vi "Actor Teardown.vi"(10 "Error":errorcluster, 11 "Self Actor in":refnum<class "Self Actor.lvclass">) -> (0 "error out":errorcluster, 2 "Teardown?":bool, 3 "Self Actor out":refnum<class "Self Actor.lvclass">)   [LabVIEW 2021, in "LVCAM.lvlib" / "Self Actor.lvclass"]
uses:
  Self Actor.lvclass
  C:/PPLs/LabVIEW-Composed-Actor-Model-LVCAM/LabVIEW-Composed-Actor-Model-LVCAM/LVCAM/LVCAM/Actor/Actor.lvclass
  Self Actor.lvclass/Self Actor.ctl
  Msgs/Actor Destroy/Actor Destroy Msg Strategy/Actor Destroy Msg Strategy.lvclass
  C:/PPLs/LabVIEW-Composed-Actor-Model-LVCAM/LabVIEW-Composed-Actor-Model-LVCAM/LVCAM/LVCAM/Msg Strategy/Msg Strategy.lvclass
  Msgs/Actor Last Ack/Actor Last Ack Msg Strategy/Actor Last Ack Msg Strategy.lvclass
  Call Msg Send.vi
  Self Msg Send.vi
  C:/PPLs/LabVIEW-Composed-Actor-Model-LVCAM/LabVIEW-Composed-Actor-Model-LVCAM/LVCAM/Msgs/Actor Create/Actor Create/Actor Create.lvclass
  C:/PPLs/LabVIEW-Composed-Actor-Model-LVCAM/LabVIEW-Composed-Actor-Model-LVCAM/LVCAM/Msgs/Actor Destroy/Actor Destroy/Actor Destroy.lvclass
  C:/PPLs/LabVIEW-Composed-Actor-Model-LVCAM/LabVIEW-Composed-Actor-Model-LVCAM/LVCAM/Msgs/Actor Last Ack/Actor Last Ack/Actor Last Ack.lvclass
  C:/PPLs/LabVIEW-Composed-Actor-Model-LVCAM/LabVIEW-Composed-Actor-Model-LVCAM/LVCAM/LVCAM/Self Actor/Self Actor.lvclass
  C:/PPLs/LabVIEW-Composed-Actor-Model-LVCAM/LabVIEW-Composed-Actor-Model-LVCAM/LVCAM/Msgs/Actor Destroy/Actor Destroy Msg Strategy/Actor Destroy Msg Strategy.lvclass
  C:/PPLs/LabVIEW-Composed-Actor-Model-LVCAM/LabVIEW-Composed-Actor-Model-LVCAM/LVCAM/Msgs/Actor Last Ack/Actor Last Ack Msg Strategy/Actor Last Ack Msg Strategy.lvclass
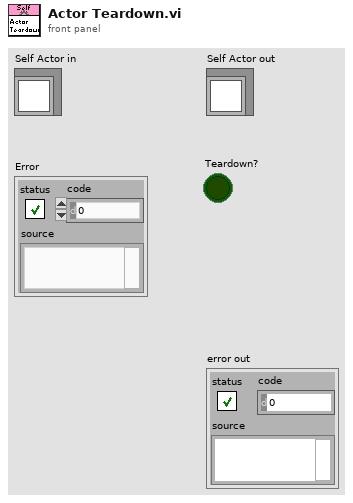
[diagram p1: front panel]
types:
  T1 = typedef "LVCAM.lvlib/Self Actor.lvclass/State.ctl" = enum16{"Msging", "Destroying"}
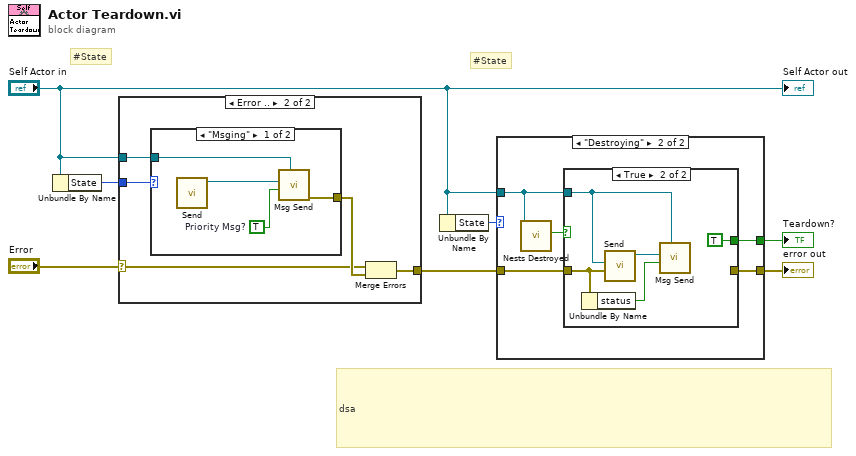
[diagram p0: block diagram]
diagram:
  # "#State"
  # "dsa"
  # "#State"
  n1 = Unbundle By Name("Self Actor in") -> ("State"=w2:T1)
  n2 = case shown="Error .." "Error" {
    selector: "Error" -> [_ w9]
    tunnel: "Self Actor in" -> [_ w12]
    tunnel: [_ w8] -> w4
    tunnel: w2 -> [_ w11]
    frame No Error {
    }
    frame Error {
      n3 = case shown="\"Msging\"" w11 {
        tunnel: w12 -> [w14 _]
        tunnel: [w13 _] -> w10
        frame "Msging" {
          w15 = TRUE  # Priority Msg?
          n4 = call "Send.vi"() -> ("Actor Destroy Msg Strategy out"=w16:refnum<class "Actor Destroy Msg Strategy.lvclass">)  [unwired: 11 in]
          n5 = call-poly "Msg Send.vi"("Actor"=w14, "Priority Msg?"=w15, "Msg"=w16) -> ("error out"=w13:errorcluster)  [unwired: 8 in]
        }
        frame "Destroying" {
          # "do nothing"
        }
      }
      n6 = Merge Errors(w9, w10) -> (w8:errorcluster)
    }
  }
  n7 = Unbundle By Name("Self Actor in") -> ("State"=w3:T1)
  n8 = case shown="\"Destroying\"" w3 {
    tunnel: [_ w22] -> w7
    tunnel: [w17 w21] -> w6
    tunnel: w4 -> [w17 w20]
    tunnel: "Self Actor in" -> [_ w19]
    frame "Msging" {
    }
    frame "Destroying" {
      n9 = call "Nests Destroyed.vi"("Self Actor in"=w19) -> ("Nests Destroyed?"=w18:bool)  [unwired: 9 in, 1 out]
      n10 = case shown="True" w18 {
        tunnel: w19 -> [_ w26]
        tunnel: w20 -> [w23 w25]
        tunnel: [_ TRUE ("Destroyed?")] -> w22
        tunnel: [w23 _] -> w21
        frame False {
        }
        frame True {
          n11 = Unbundle By Name(w25) -> ("status"=w24:bool)
          n12 = call "Send.vi"("Nest Error"=w25, "Nest Actor"=w26) -> ("Actor Last Ack Msg Strategy out"=w27:refnum<class "Actor Last Ack Msg Strategy.lvclass">)  [unwired: 9 in]
          n13 = call-poly "Msg Send.vi"("Actor"=w26, "Priority Msg?"=w24, "Msg"=w27) -> ()  [unwired: 8 in, 1 out]
        }
      }
    }
  }
  "Teardown?" <- w7
  "error out" <- w6
  "Self Actor out" <- "Self Actor in"
